vi "ReadCapacitanceBuffers.vi"(8 "error in (no error)":errorcluster, 10 "Status":refnum<vi>, 11 "VISA Refnum in":refnum<visa-resource-name>) -> (0 "error out":errorcluster, 3 "CapacitanceInfos":T1[](array[typedef]))   [LabVIEW 2020]
uses:
  CapacitanceRecord.ctl
  Keithley 2600 Series/Keithley 2600 Series.lvlib
panel:
  out "Array":string[](array[string])
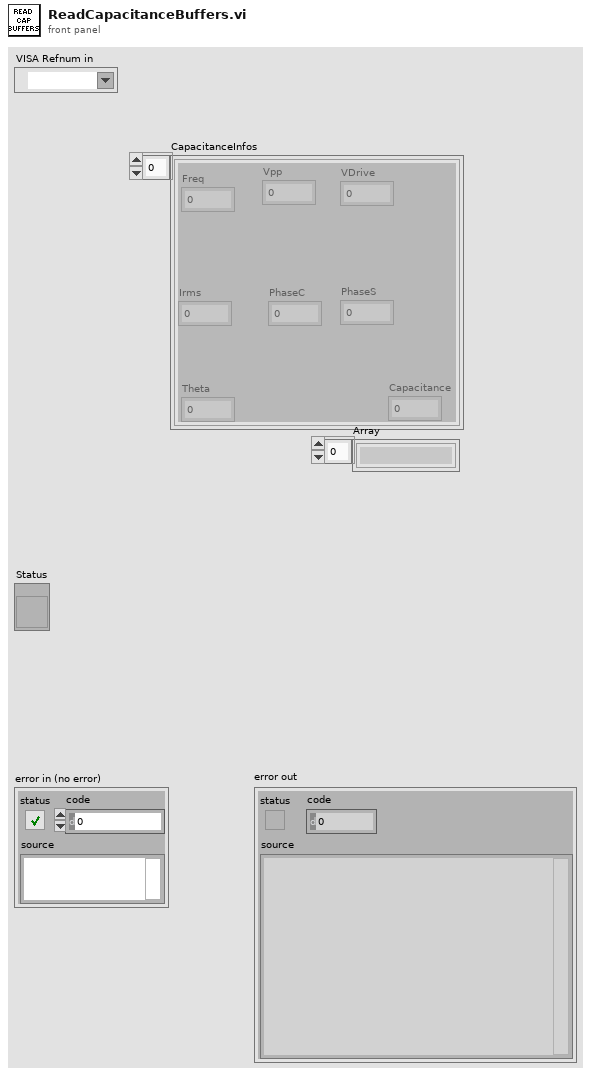
[diagram p1: front panel]
types:
  T1 = typedef "CapacitanceRecord.ctl" = cluster{"Freq":dbl, "Vpp":dbl, "PhaseS":dbl, "Irms":dbl, "PhaseC":dbl, "Theta":dbl, "VDrive":dbl, "Capacitance":dbl}
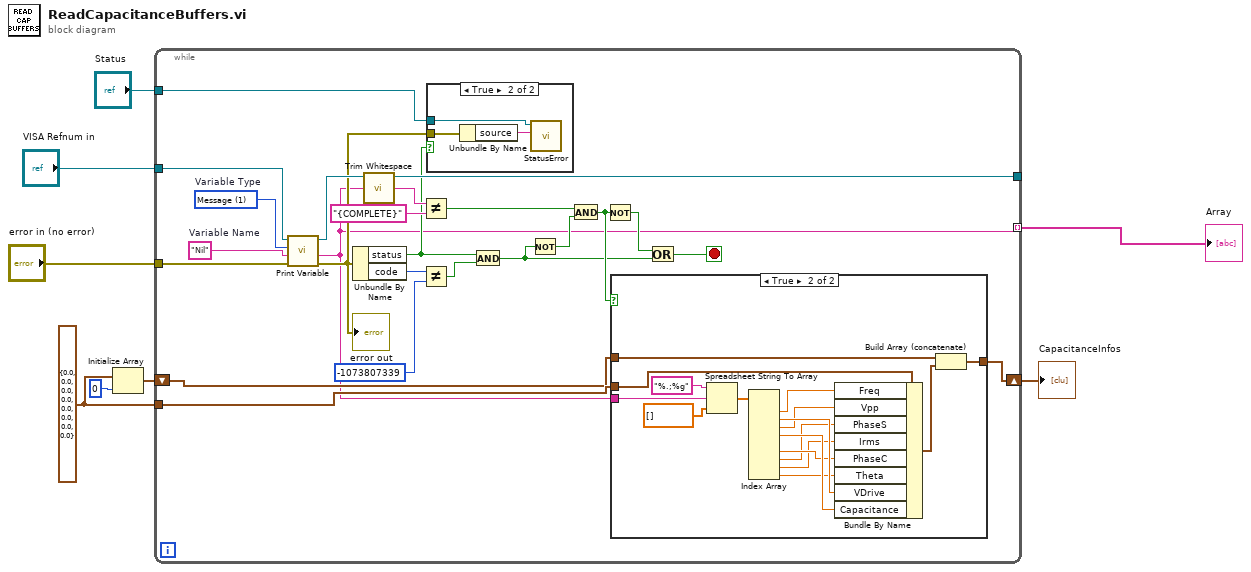
[diagram p0: block diagram]
diagram:
  w3 = T1 {"Freq"=0.0, "Vpp"=0.0, "PhaseS"=0.0, "Irms"=0.0, "PhaseC"=0.0, "Theta"=0.0, "VDrive"=0.0, "Capacitance"=0.0} ("cluster")
  n1 = Initialize Array(w3, 0 ("dimension size")) -> (w2:T1[])
  n2 = while {
    tunnel: "VISA Refnum in" -> [w29]
    tunnel: "error in (no error)" -> [w28]
    tunnel: [w27] -> _
    shift-right: [w19] -> w4
    shift-left: w2 -> [w17]
    tunnel: "Status" -> [w20]
    tunnel: w3 -> [w18]
    tunnel: [w9] -> w1 mode=indexing
    stop <- w22 stop-if-true
    w31 = 1 items=["Number", "Message"]  # Variable Type
    w30 = "Nil"  # Variable Name
    n3 = call "Print Variable.vi"("error in (no error)"=w28, "Variable Name"=w30, "Variable Type (0: Number)"=w31, "VISA resource name"=w29) -> ("error out"=w21:errorcluster, "Message"=w9:string, "VISA resource name out"=w27:refnum<visa-resource-name>)  [unwired: 4 in, 1 out]
    "error out" <- w21
    n4 = Unbundle By Name(w21) -> ("status"=w16:bool, "code"=w15:i32)
    n5 = call <vilib>:"Trim Whitespace.vi"("string"=w9) -> ("trimmed string"=w26:string)  [unwired: 1 in]
    n6 = Not Equal?(x=w26, y="{COMPLETE}") -> (x != y?=w24:bool)
    n7 = Not Equal?(x=w15, y=-1073807339) -> (x != y?=w13:bool)
    n8 = case shown="True" w16 {
      tunnel: w21 -> [_ w33]
      tunnel: w20 -> [_ w32]
      frame False {
      }
      frame True {
        n9 = Unbundle By Name(w33) -> ("source"=w34:string)
        n10 = call "StatusError.vi"("Text.Text"=w34, "String in"=w32) -> ()  [unwired: 10 in]
      }
    }
    n11 = And(x=w16, y=w13) -> (x .and. y?=w11:bool)
    n12 = Not(x=w11) -> (.not. x?=w10:bool)
    n13 = And(x=w24, y=w10) -> (x .and. y?=w12:bool)
    n14 = Not(x=w12) -> (.not. x?=w23:bool)
    n15 = case shown="True" w12 {
      tunnel: w9 -> [_ w49]
      tunnel: w17 -> [w35 w48]
      tunnel: [w35 w47] -> w19
      tunnel: w18 -> [_ w46]
      frame False {
      }
      frame True {
        n16 = Spreadsheet String To Array(format string="%.;%g", spreadsheet string=w49, array type (2D Dbl)=dbl[] []) -> (array=w44:dbl[])  [unwired: 1 in]
        n17 = Index Array(array=w44) -> (element #1=w43:dbl, element #2=w42:dbl, element #3=w41:dbl, element #4=w40:dbl, element #6=w39:dbl, element #7=w38:dbl, element #8=w37:dbl, element #9=w36:dbl)  [unwired: 9 in, 1 out]
        n18 = Bundle By Name(cluster=w46, "Freq"=w43, "Vpp"=w41, "PhaseS"=w38, "Irms"=w37, "PhaseC"=w39, "Theta"=w36, "VDrive"=w42, "Capacitance"=w40) -> (w45:T1)
        n19 = Build Array (concatenate)(w48, w45) -> (w47:T1[])
      }
    }
    n20 = Or(x=w23, y=w11) -> (x .or. y?=w22:bool)
  }
  "CapacitanceInfos" <- w4
  "Array" <- w1
